vi "Autolab Complete Example (A).vi"() -> ()   [LabVIEW 2011]
uses:
  C:/Program Files/Metrohm Autolab/Autolab SDK 1.10/EcoChemie.Autolab.Sdk.dll
  EcoChemie.Autolab.Sdk.dll
panel:
  out "PotentialApplied":dbl
  in  "Abort":bool
  in  "fileName":string
  out "IsMeasuring":bool
  in  "Save":bool
  in  "start measure":bool
  in  "Stop":bool
  out "Value Y":dbl
  out "Value X":dbl
  out "XY Graph 2":cluster{"Y":dbl[], "Y":dbl[]}[](graph)
  in  "Signal X":string(combo)
  in  "Signal Y":string(combo)
  out "Setpoint":dbl
  out "Mode":i32(ring) items=["Potentiostatic", "Galvanostatic"]
  out "CurrentRange":i32(ring) items=["CR07_1A"=0, "CR06_10A"=1, "CR01_100A"=2, "CR00_1000A"=3, "CR05_20A"=20, "CR04_40A"=40, "CR03_50A"=60, "CR02_80A"=80, "CR19_1pA"=-12, "CR18_10pA"=-11, "CR17_100pA"=-10, "CR16_1nA"=-9, "CR15_10nA"=-8, "CR14_100nA"=-7, "CR13_1uA"=-6, "CR12_10uA"=-5, "CR11_100uA"=-4, "CR10_1mA"=-3, "CR09_10mA"=-2, "CR08_100mA"=-1]
  out "Bandwidth":i32(ring) items=["UltraHigh_Speed", "High_Speed", "High_Stability"]
  out "error out":errorcluster
  in  "Procedure":path=path "Standard Nova Procedures/Cyclic voltammetry.nox"
  in  "Load":bool
  in  "Hardware Setup File":path
  out "EI status supported for":string[](array[string])
  out "Oscillation":bool
  in  "Channel":i32(ring) items=["16"=15, "15"=14, "14"=13, "13"=12, "12"=11, "11"=10, "10"=9, "9"=8, "8"=7, "7"=6, "6"=5, "5"=4, "4"=3, "3"=2, "2"=1, "1"=0]
  out "IsConnected":bool
  out "Sample":dbl
  in  "usPerLoop 2":u16=20000
  in  "usPerLoop":u16=20000
  in  "Sampler Type":T1(ring)
  in  "Loops 2":i32=1 min=1
  in  "Loops":i32=1 min=1
  in  "Gain 2":i32(ring) items=["Gain_1"=0, "Gain_10"=64, "Gain_100"=128, "Gain_1000"=192]
  in  "Gain":i32(ring) items=["Gain_1"=0, "Gain_10"=64, "Gain_100"=128, "Gain_1000"=192]
  out "DIO Status P2 R":bool[](array[boolean])
  in  "DIO Status P2 W":bool[](array[boolean])
  in  "Port P2":i32(ring) items=["Port_A", "Port_B", "Port_C"]
  in  "P2 Direction":enum16{"Input(read)", "Output(write)"}(ring)
  out "DIO Status P1 R":bool[](array[boolean])
  in  "Port P1":i32(ring) items=["Port_A", "Port_B", "Port_C"]
  in  "P1 Direction":enum16{"Input(read)", "Output(write)"}(ring)
  in  "DIO Status P1 W":bool[](array[boolean])
  in  "voltage":dbl
  in  "channel":i32 min=0 max=16
  out "Value":dbl
  in  "Signal List":string(combo)
  out "Current":dbl
  out "Potential":dbl
  out "PotentialOverload":bool
  out "TemperatureOverload":bool
  out "CurrentOverload":bool
  out "ManualCellSwitch":bool
  out "Cell":bool
  in  "Setpoint":dbl
  in  "Current Range":i32(ring)=-3 items=["CR07_1A"=0, "CR06_10A"=1, "CR01_100A"=2, "CR00_1000A"=3, "CR05_20A"=20, "CR04_40A"=40, "CR03_50A"=60, "CR02_80A"=80, "CR19_1pA"=-12, "CR18_10pA"=-11, "CR17_100pA"=-10, "CR16_1nA"=-9, "CR15_10nA"=-8, "CR14_100nA"=-7, "CR13_1uA"=-6, "CR12_10uA"=-5, "CR11_100uA"=-4, "CR10_1mA"=-3, "CR09_10mA"=-2, "CR08_100mA"=-1]
  in  "Cell On/Off":i32(ring) items=["Off", "On"]
  in  "Bandwidth":i32(ring)=2 items=["UltraHigh_Speed", "High_Speed", "High_Stability"]
  in  "Mode":i32(ring) items=["Potentiostatic", "Galvanostatic"]
  in  "Embedded Exe File":path
  # "Create Autolab"
  # "Measuring"
  # "Electrochemical Interface"
  # "ADC"
  # "DIO"
  # "DAC"
  # "Sampler Signals"
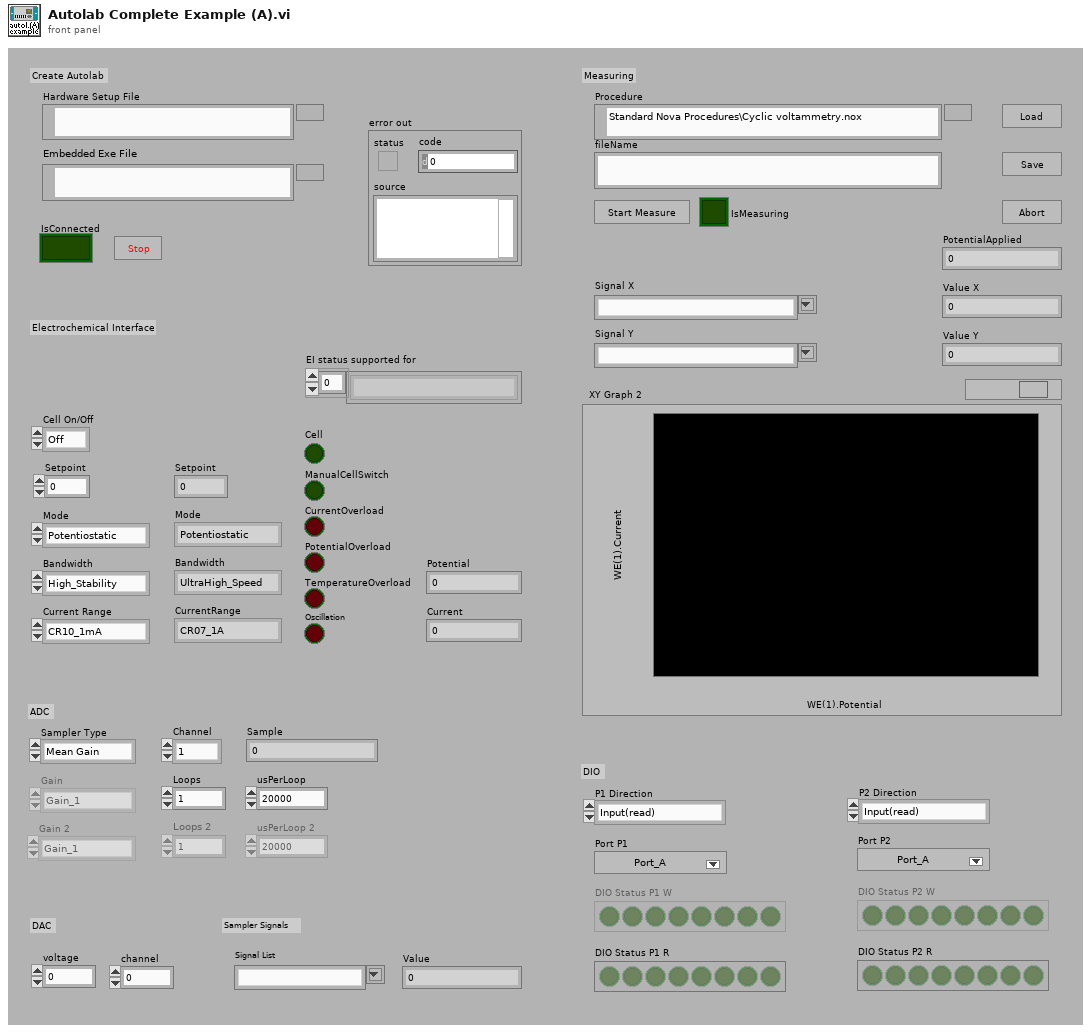
[diagram p1: front panel]
types:
  T1 = enum16{"Mean Gain", "Mean Fixed", "One Fixed", "One Gain"}
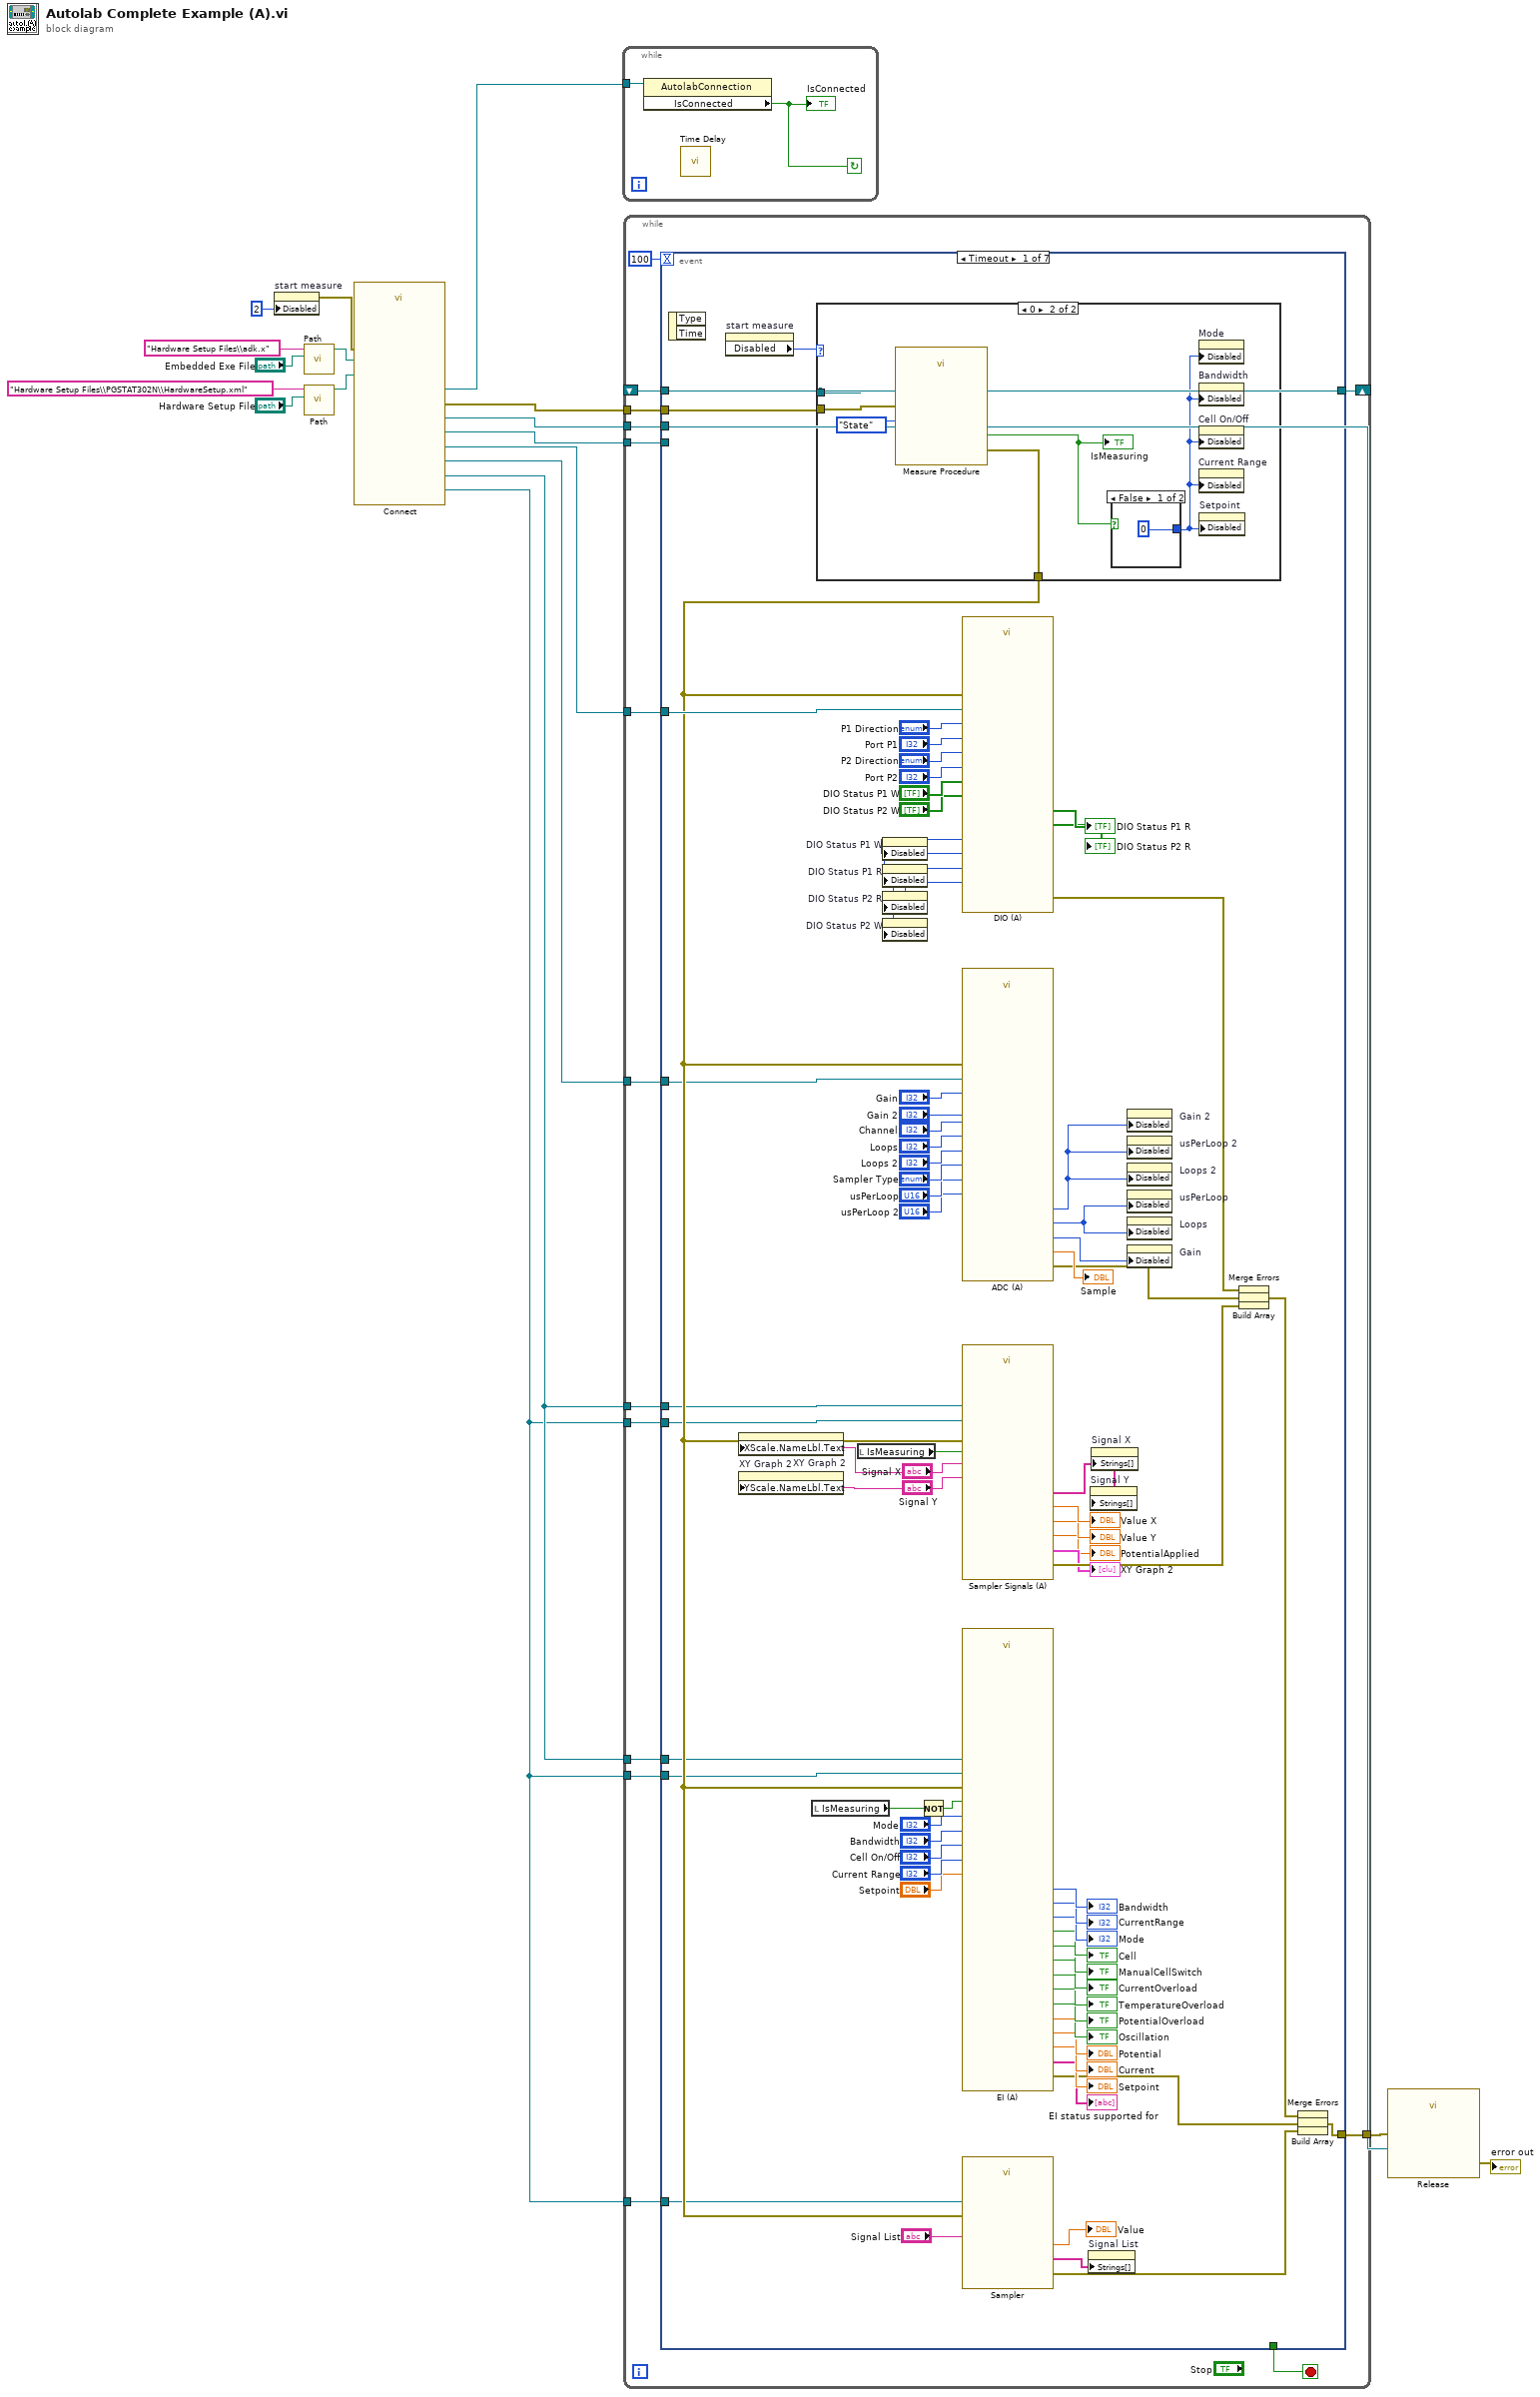
[diagram p0: block diagram]
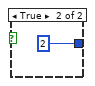
[diagram p3: hidden frame]
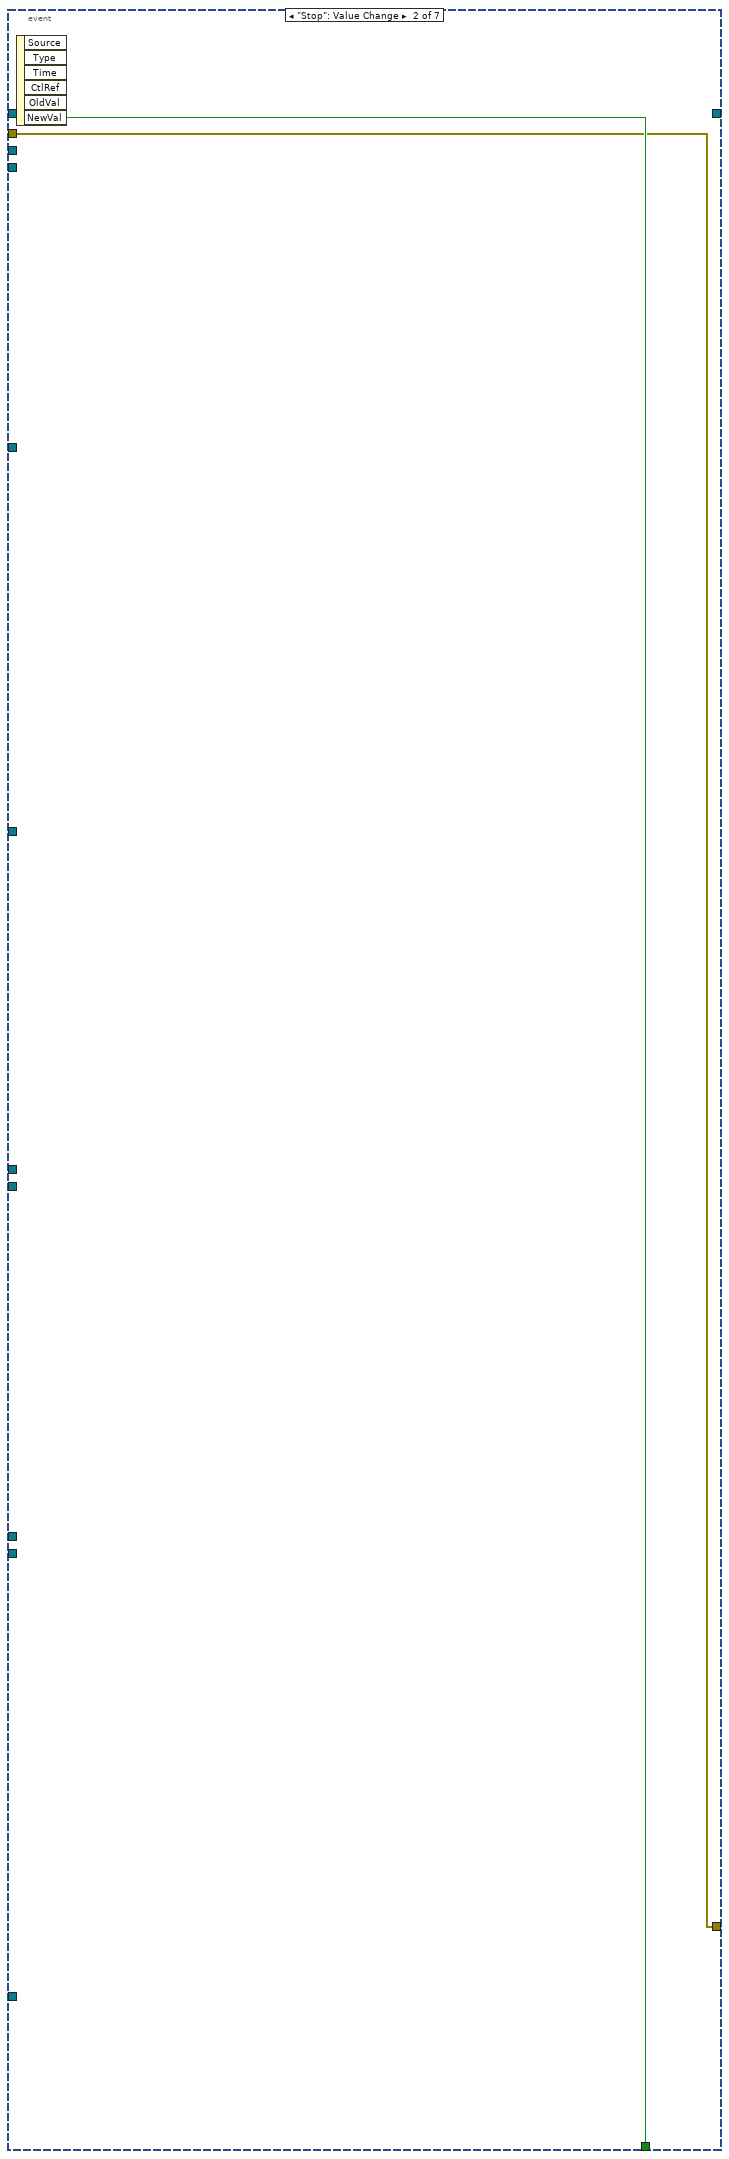
[diagram p4: hidden frame]
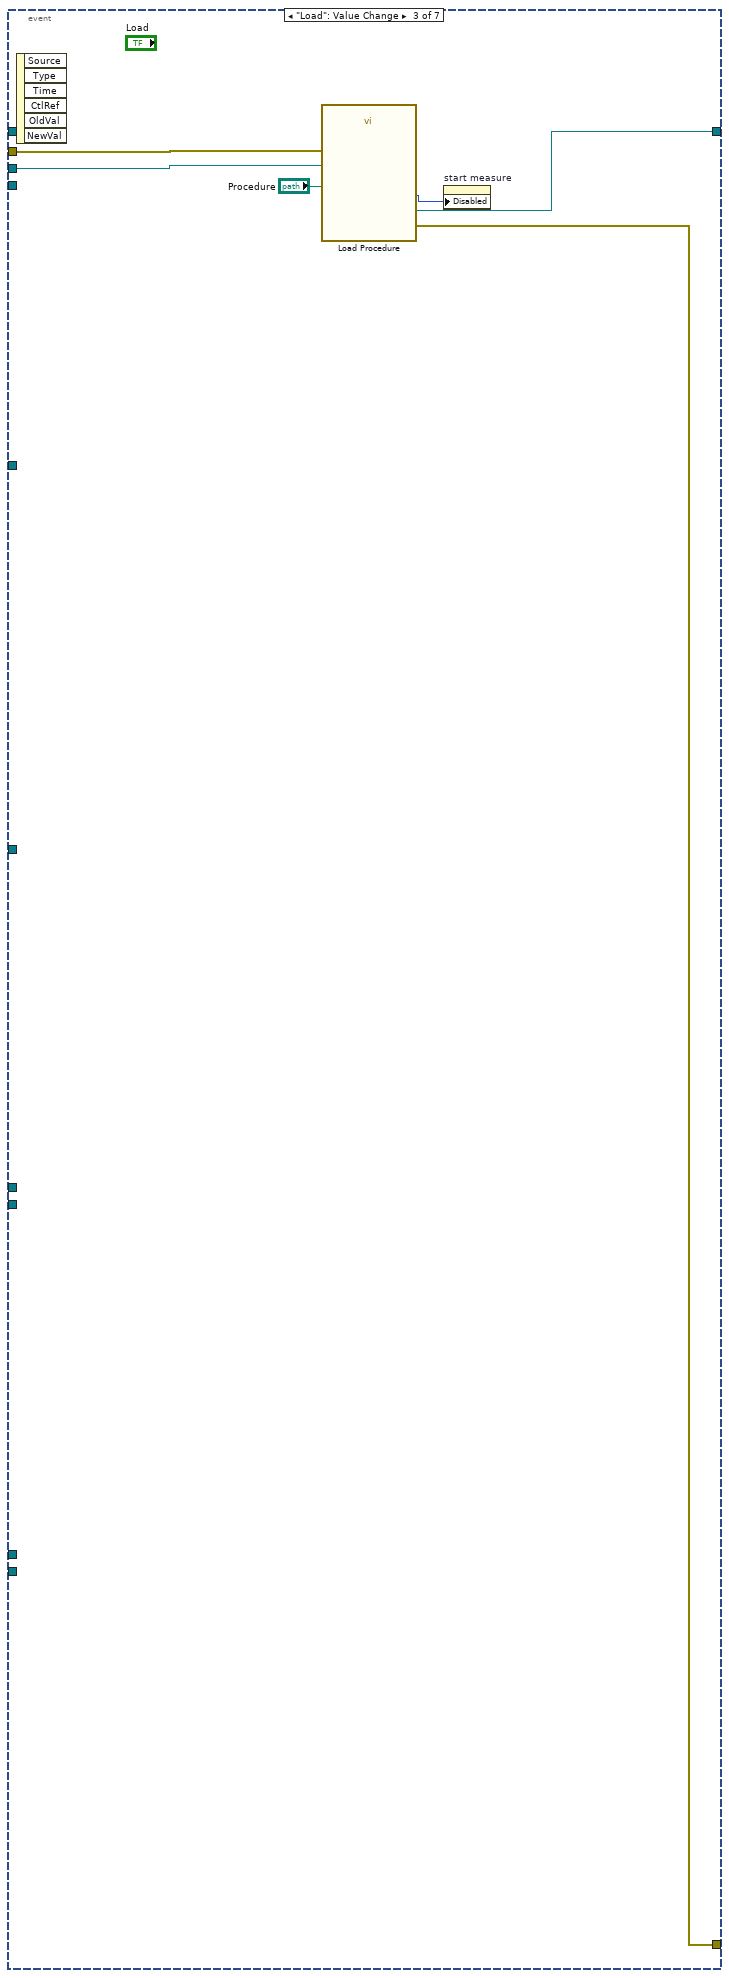
[diagram p5: hidden frame]
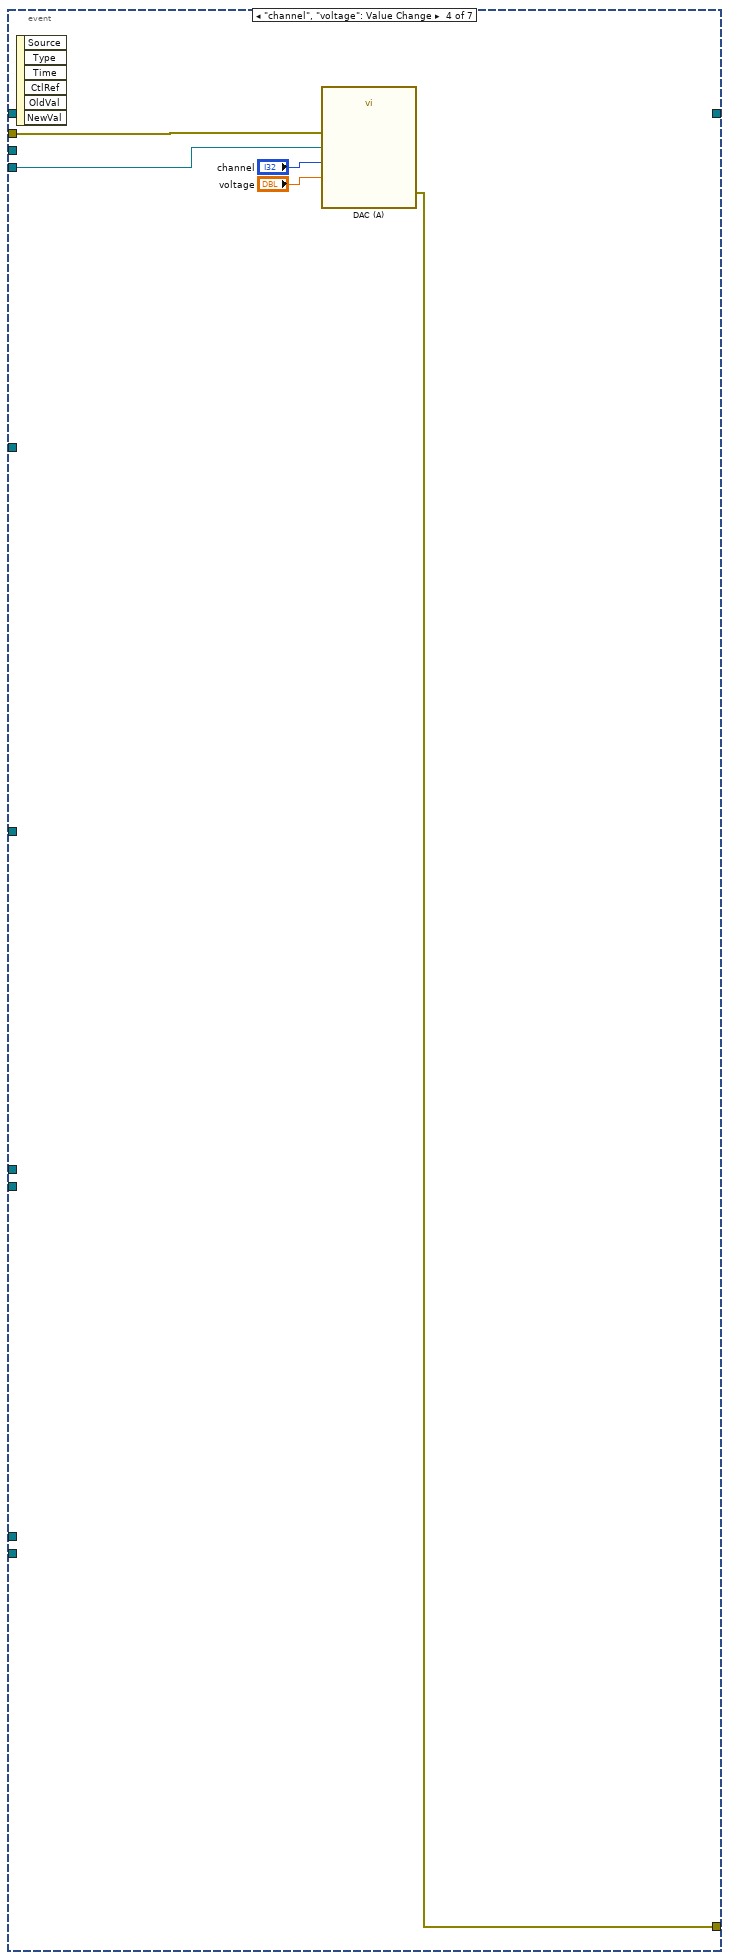
[diagram p6: hidden frame]
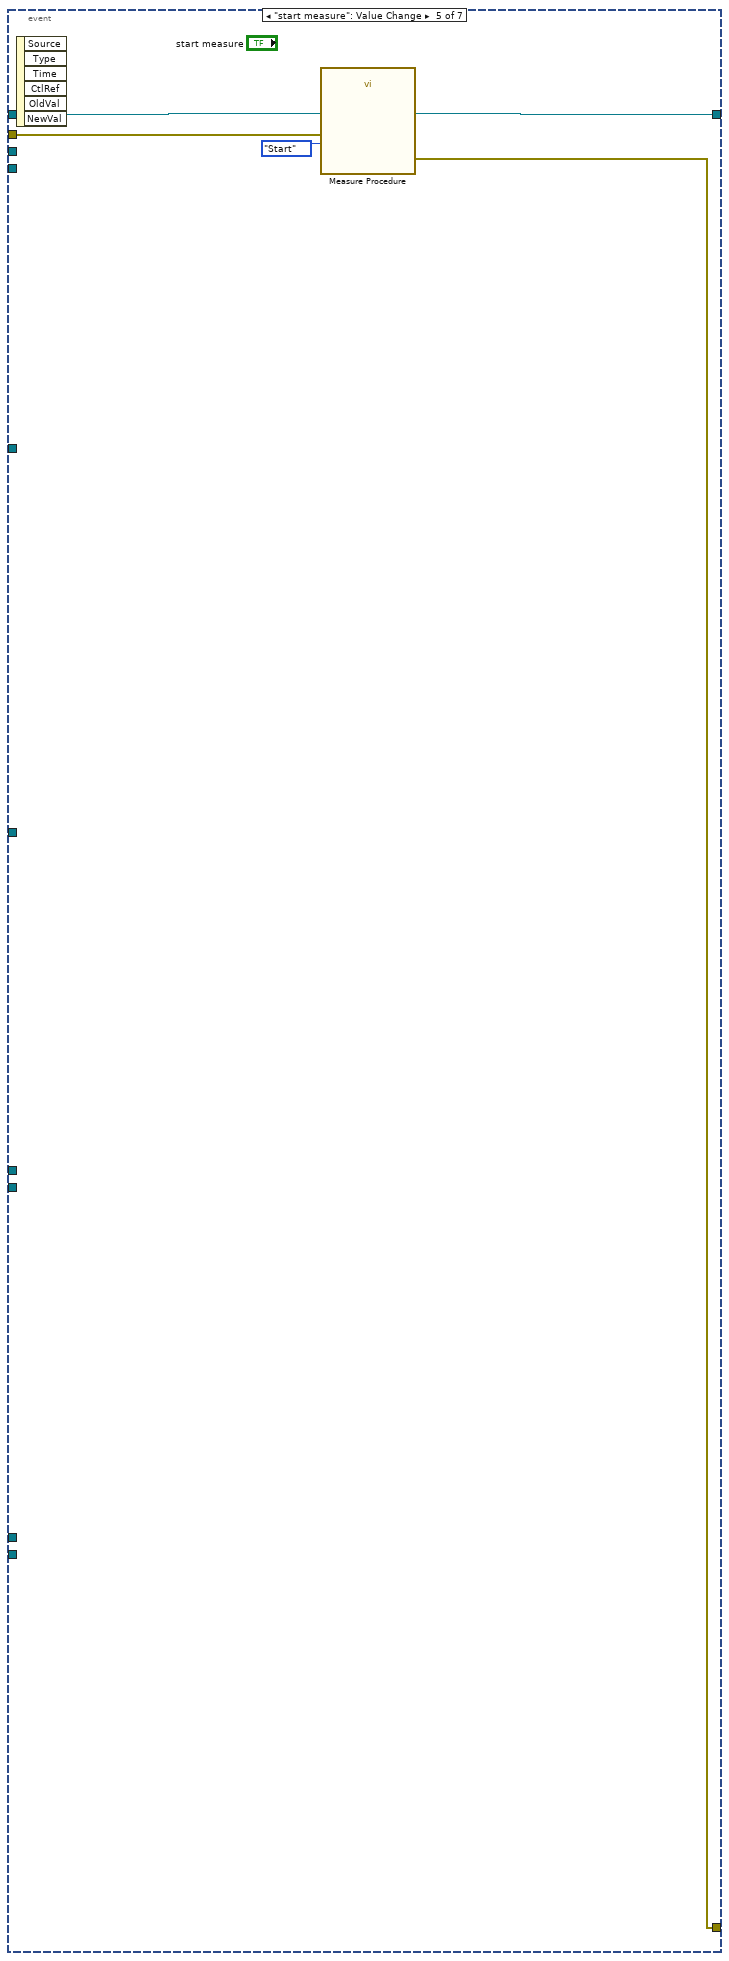
[diagram p7: hidden frame]
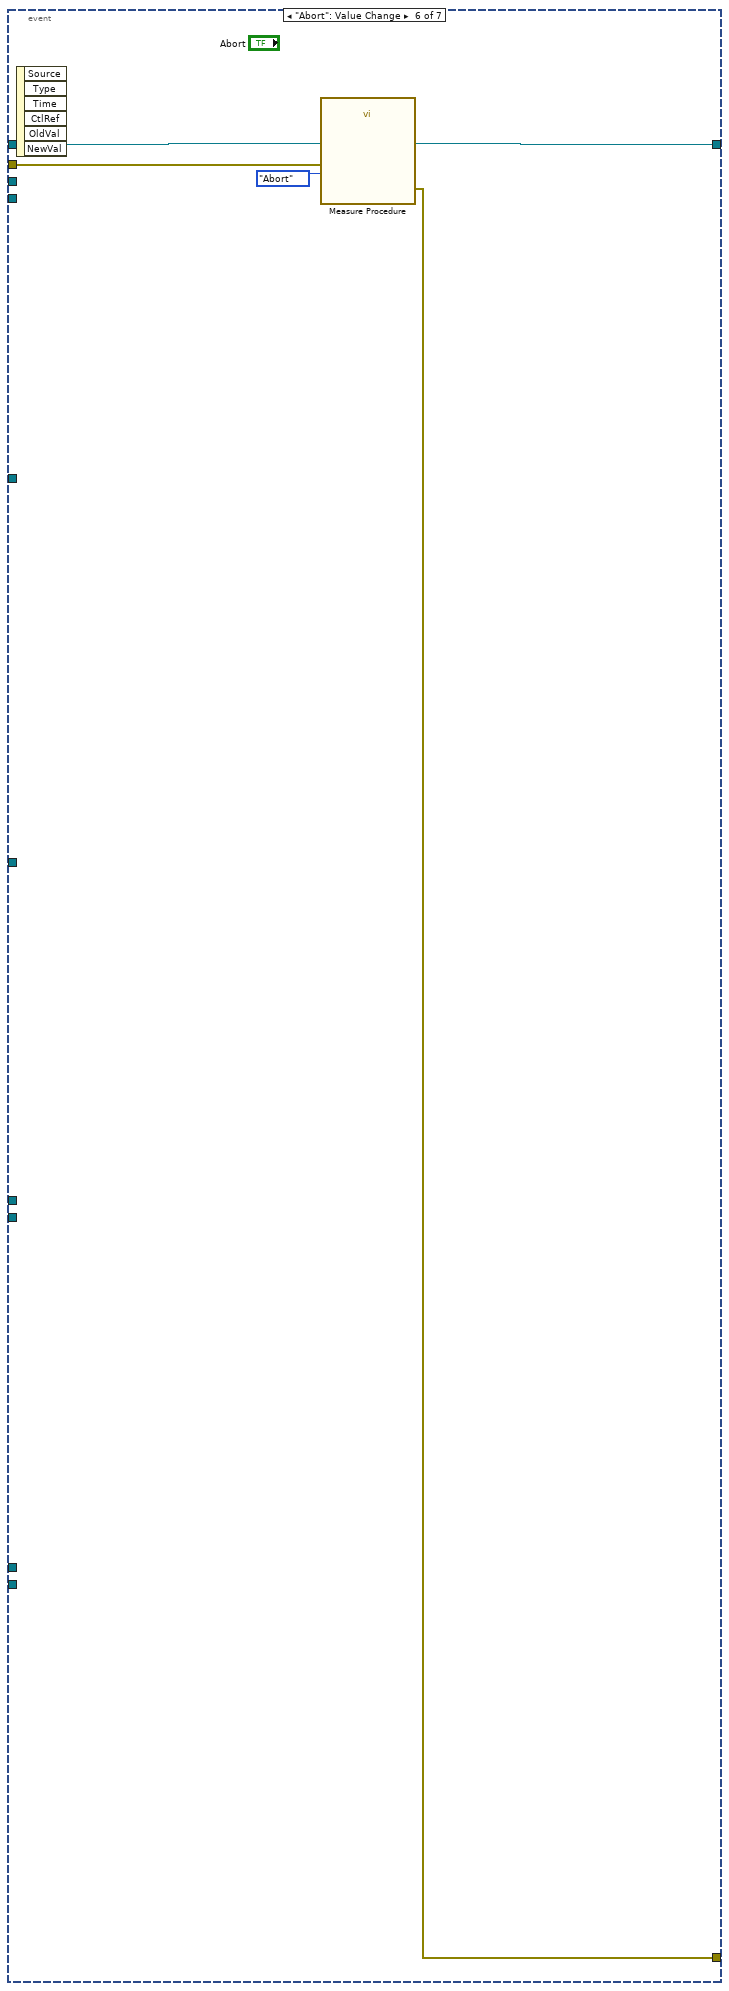
[diagram p8: hidden frame]
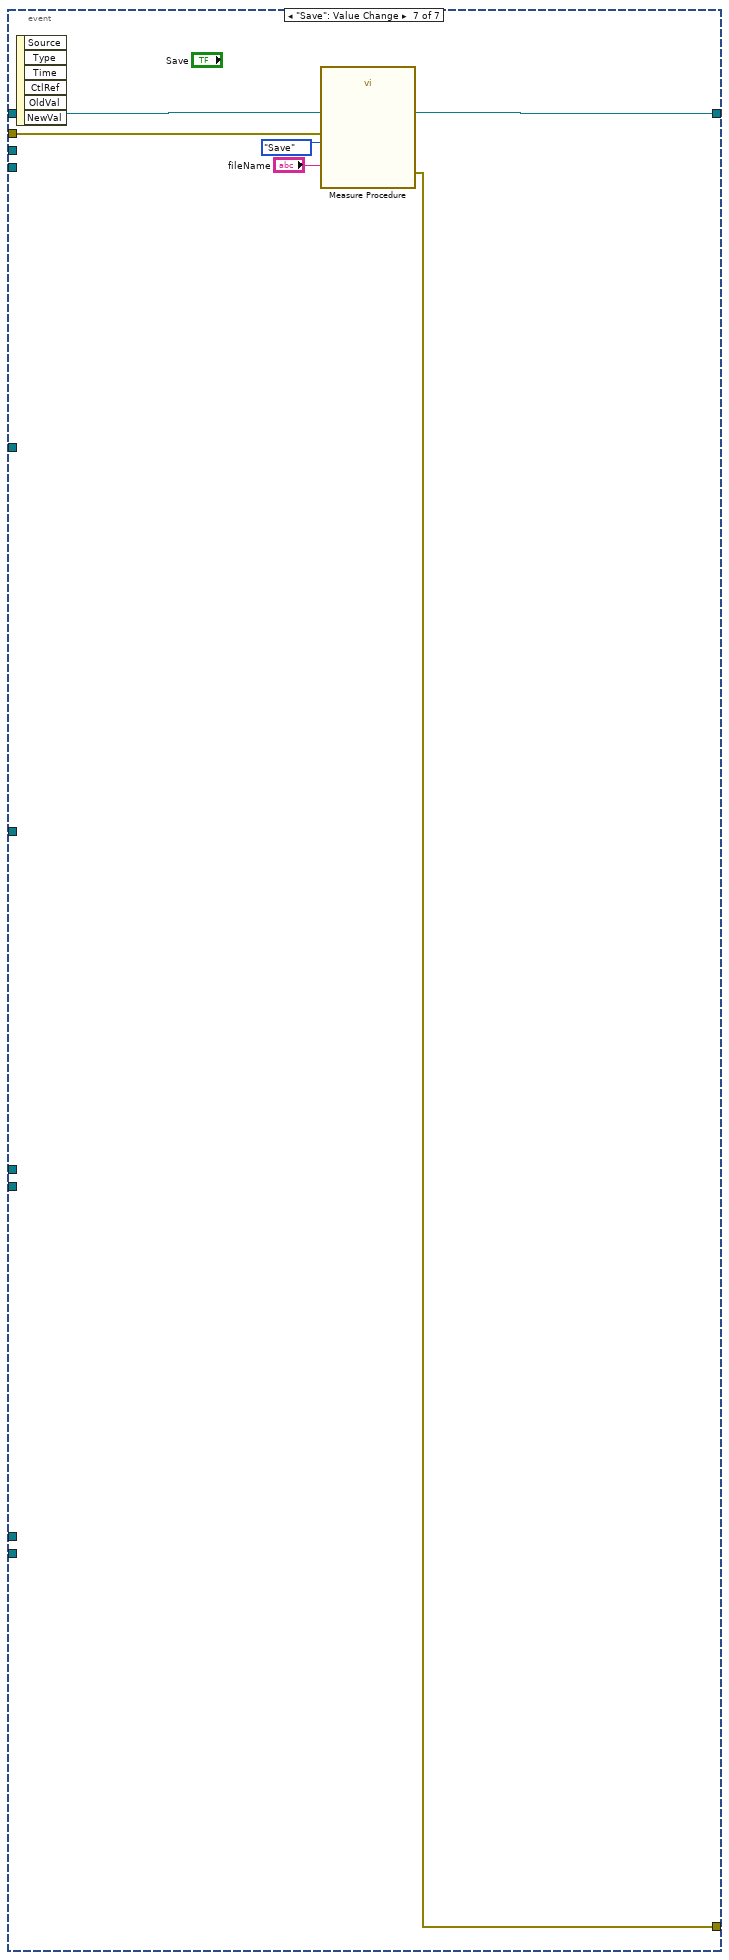
[diagram p9: hidden frame]
diagram:
  n1 = property on="start measure" class="Bool"("Disabled"=u8 2) -> (error out=w2:errorcluster)  [unwired: 2 in, 1 out]
  n2 = call "Path.vi"("File"="Embedded Exe File", "name or relative path"="Hardware Setup Files\\adk.x") -> ("appended path"=w5:path)  [unwired: 9 in]
  n3 = call "Path.vi"("File"="Hardware Setup File", "name or relative path"="Hardware Setup Files\\PGSTAT302N\\HardwareSetup.xml") -> ("appended path"=w6:path)  [unwired: 9 in]
  n4 = call "Connect.vi"("Embedded Exe File"=w5, "Hardware Setup File"=w6, "error in (no error)"=w2) -> ("Adc"=w13:refnum<k24>, "Dac"=w15:refnum<k24>, "Dio"=w14:refnum<k24>, "Sampler"=w11:refnum<k24>, "AutolabConnection"=w17:refnum<k24>, "instrument"=w9:refnum<k24>, "Ei"=w12:refnum<k24>, "error out"=w16:errorcluster)  [unwired: 5 in]
  n5 = while {
    tunnel: w17 -> [w20]
    stop <- w19 continue-if-true
    n6 = property class="AutolabConnection"(reference=w20) -> ("IsConnected"=w19:bool)  [unwired: 1 in, 2 out]
    "IsConnected" <- w19
    n7 = call "Time Delay"() -> ()  [unwired: 11 in, 1 out]
  }
  n8 = while {
    shift-right: [w32] -> _
    shift-left: _ -> [w33]
    tunnel: w16 -> [w31]
    tunnel: w9 -> [w30]
    tunnel: w15 -> [w29]
    tunnel: w14 -> [w28]
    tunnel: w13 -> [w27]
    tunnel: w11 -> [w26]
    tunnel: w12 -> [w25]
    tunnel: w11 -> [w24]
    tunnel: w11 -> [w23]
    tunnel: w12 -> [w22]
    tunnel: [w21] -> w10
    stop <- w35 stop-if-true
    n9 = event shown="[0] Timeout" {
      selector: _ -> [_ _ _ _ _ _ _]
      dyn-events: _ -> [_ _ _ _ _ _ _]
      timeout: 100 -> [_ _ _ _ _ _ _]
      tunnel: [_ w121 _ _ _ _ _] -> w35
      tunnel: w33 -> [w46 _ _ _ w135 w139 w143]
      tunnel: [w46 _ w125 _ w135 w139 w143] -> w32
      tunnel: w31 -> [w62 w120 w124 w129 w134 w138 w142]
      tunnel: w30 -> [_ _ w123 _ _ _ _]
      tunnel: w29 -> [_ _ _ w130 _ _ _]
      tunnel: w28 -> [w63 _ _ _ _ _ _]
      tunnel: w27 -> [w60 _ _ _ _ _ _]
      tunnel: w26 -> [w59 _ _ _ _ _ _]
      tunnel: w25 -> [w58 _ _ _ _ _ _]
      tunnel: w24 -> [w57 _ _ _ _ _ _]
      tunnel: w23 -> [w56 _ _ _ _ _ _]
      tunnel: w22 -> [w55 _ _ _ _ _ _]
      tunnel: [w48 w120 w122 w128 w133 w137 w141] -> w21
      event Timeout {
        n10 = event-data() -> ()  [unwired: 1 in, 2 out]
        n11 = property on="start measure" class="Bool"() -> ("Disabled"=w64:u8)  [unwired: 2 in, 2 out]
        n12 = property on="XY Graph 2" class="XYGraph (strict)"("XScale.NameLbl.Text"="Signal X") -> ()  [unwired: 2 in, 2 out]
        n13 = property on="XY Graph 2" class="XYGraph (strict)"("YScale.NameLbl.Text"="Signal Y") -> ()  [unwired: 2 in, 2 out]
        n14 = local read "IsMeasuring"() -> (w47:bool)
        n15 = case shown="0" w64 {
          tunnel: w46 -> [_ w114]
          tunnel: w62 -> [w111 w113]
          tunnel: [w111 w112] -> w61
          frame 2, Default {
          }
          frame 0 {
            n16 = call "Measure Procedure.vi"("error in"=w113, "Request for procedure"=enum16{"State", "Save", "Abort", "Start"}."State", "LoadProcedure"=w114) -> ("error out"=w112:errorcluster, "IsMeasuring"=w116:bool)  [unwired: 7 in]
            "IsMeasuring" <- w116
            n17 = case shown="False" w116 {
              tunnel: [u8 0 ("Disabled") u8 2 ("Disabled")] -> w117
              frame False {
              }
              frame True {
              }
            }
            n18 = property on="Mode" class="Ring (strict)"("Disabled"=w117) -> ()  [unwired: 2 in, 2 out]
            n19 = property on="Bandwidth" class="Ring (strict)"("Disabled"=w117) -> ()  [unwired: 2 in, 2 out]
            n20 = property on="Cell On/Off" class="Ring (strict)"("Disabled"=w117) -> ()  [unwired: 2 in, 2 out]
            n21 = property on="Current Range" class="Ring (strict)"("Disabled"=w117) -> ()  [unwired: 2 in, 2 out]
            n22 = property on="Setpoint" class="DigNum (strict)"("Disabled"=w117) -> ()  [unwired: 2 in, 2 out]
          }
        }
        n23 = local read "IsMeasuring"() -> (w43:bool)
        n24 = Not(x=w47) -> (.not. x?=w110:bool)
        n25 = call "DIO (A).vi"("Dio"=w63, "DIO Status P1 W"="DIO Status P1 W", "DIO Status P2 W"="DIO Status P2 W", "error in (no error)"=w61, "Port P1"="Port P1", "Port P2"="Port P2", "P1 Direction"="P1 Direction", "P2 Direction"="P2 Direction") -> ("Disable P1 W"=w80:u8, "Disable P2 W"=w77:u8, "DIO Status P1 R"=→"DIO Status P1 R":bool[], "Disable P1 R"=w79:u8, "DIO Status P2 R"=→"DIO Status P2 R":bool[], "Disable P2 R"=w78:u8, "error out"=w54:errorcluster)  [unwired: 5 in]
        n26 = property on="DIO Status P1 W" class="Arr (strict)"("Disabled"=w80) -> ()  [unwired: 2 in, 2 out]
        n27 = property on="DIO Status P1 R" class="Arr (strict)"("Disabled"=w79) -> ()  [unwired: 2 in, 2 out]
        n28 = property on="DIO Status P2 R" class="Arr (strict)"("Disabled"=w78) -> ()  [unwired: 2 in, 2 out]
        n29 = property on="DIO Status P2 W" class="Arr (strict)"("Disabled"=w77) -> ()  [unwired: 2 in, 2 out]
        n30 = call "ADC (A).vi"("Adc"=w60, "Loops 2"="Loops 2", "Gain"="Gain", "Loops"="Loops", "Sampler Type"="Sampler Type", "Gain 2"="Gain 2", "usPerLoop 2"="usPerLoop 2", "error in"=w61, "Channel"="Channel", "usPerLoop"="usPerLoop") -> ("Sample"=→"Sample":dbl, "Disable MeanGain"=w67:u8, "Disable MeanFixed"=w65:u8, "Disable OneFixed"=w66:u8, "error out"=w53:errorcluster)  [unwired: 1 in]
        n31 = call "Sampler Signals (A).vi"("IsMeasuring"=w43, "EI"=w55, "Sampler"=w59, "Signal X"="Signal X", "Signal Y"="Signal Y", "error in"=w61) -> ("PotentialApplied"=→"PotentialApplied":dbl, "X"=→"Value X":dbl, "Y"=→"Value Y":dbl, "XY Graph"=→"XY Graph 2":cluster{"Y":dbl[], "Y":dbl[]}[], "GetSignals"=w42:string[], "error out"=w52:errorcluster)  [unwired: 4 in]
        n32 = call "EI (A).vi"("Sampler"=w57, "Ei"=w58, "CellOnOff"="Cell On/Off", "Setpoint"="Setpoint", "Bandwidth"="Bandwidth", "CurrentRange"="Current Range", "Mode"="Mode", "error in (no error)"=w61, "Disable Sampler"=w110) -> ("Cell"=→"Cell":bool, "PotentialOverload"=→"PotentialOverload":bool, "ManualCellSwitch"=→"ManualCellSwitch":bool, "TemperatureOverload"=→"TemperatureOverload":bool, "CurrentOverload"=→"CurrentOverload":bool, "Oscillation"=→"Oscillation":bool, "Setpoint"=→"Setpoint":dbl, "Bandwidth"=→"Bandwidth":i32, "CurrentRange"=→"CurrentRange":i32, "Mode"=→"Mode":i32, "EI status supported for"=→"EI status supported for":string[], "Potential"=→"Potential":dbl, "Current"=→"Current":dbl, "error out"=w50:errorcluster)  [unwired: 5 in]
        n33 = call "Sampler.vi"("error in (no error)"=w61, "Signal List"="Signal List", "Sampler"=w56) -> ("error out"=w51:errorcluster, "Signal Value"=→"Value":dbl, "GetSignals"=w90:string[])  [unwired: 6 in]
        n34 = property on="Signal List" class="CmbBox"("Strings[]"=w90) -> ()  [unwired: 2 in, 2 out]
        n35 = property on="Signal Y" class="CmbBox"("Strings[]"=w42) -> ()  [unwired: 2 in, 2 out]
        n36 = property on="Signal X" class="CmbBox"("Strings[]"=w42) -> ()  [unwired: 2 in, 2 out]
        n37 = property on="Gain 2" class="Ring (strict)"("Disabled"=w65) -> ()  [unwired: 2 in, 2 out]
        n38 = property on="usPerLoop 2" class="DigNum (strict)"("Disabled"=w65) -> ()  [unwired: 2 in, 2 out]
        n39 = property on="Loops 2" class="DigNum (strict)"("Disabled"=w65) -> ()  [unwired: 2 in, 2 out]
        n40 = property on="usPerLoop" class="DigNum (strict)"("Disabled"=w67) -> ()  [unwired: 2 in, 2 out]
        n41 = property on="Loops" class="DigNum (strict)"("Disabled"=w67) -> ()  [unwired: 2 in, 2 out]
        n42 = property on="Gain" class="Ring (strict)"("Disabled"=w66) -> ()  [unwired: 2 in, 2 out]
        n43 = Build Array(w54, w53, w52) -> (w36:errorcluster[])
        n44 = Merge Errors(w36) -> (w49:errorcluster)
        n45 = Build Array(w49, w50, w51) -> (w37:errorcluster[])
        n46 = Merge Errors(w37) -> (w48:errorcluster)
      }
      event "Stop": Value Change {
        n47 = event-data() -> ("NewVal"=w121:bool)  [unwired: 1 in, 5 out]
      }
      event "Load": Value Change {
        n48 = event-data() -> ()  [unwired: 1 in, 6 out]
        n49 = call "Load Procedure.vi"("error in (no error)"=w124, "Procedure"="Procedure", "Instrument"=w123) -> ("error out"=w122:errorcluster, "Numeric"=w127:i32, "LoadProcedure"=w125:refnum<k24>)  [unwired: 5 in, 1 out]
        n50 = property on="start measure" class="Bool"("Disabled"=w127) -> ()  [unwired: 2 in, 2 out]
      }
      event "channel", "voltage": Value Change {
        n51 = event-data() -> ()  [unwired: 1 in, 6 out]
        n52 = call "DAC (A).vi"("error in (no error)"=w129, "voltage"="voltage", "channel"="channel", "Dac"=w130) -> ("error out"=w128:errorcluster)  [unwired: 7 in]
      }
      event "start measure": Value Change {
        n53 = event-data() -> ()  [unwired: 1 in, 6 out]
        n54 = call "Measure Procedure.vi"("error in"=w134, "Request for procedure"=enum16{"State", "Save", "Abort", "Start"}."Start", "LoadProcedure"=w135) -> ("error out"=w133:errorcluster)  [unwired: 7 in, 1 out]
      }
      event "Abort": Value Change {
        n55 = event-data() -> ()  [unwired: 1 in, 6 out]
        n56 = call "Measure Procedure.vi"("error in"=w138, "Request for procedure"=enum16{"State", "Save", "Abort", "Start"}."Abort", "LoadProcedure"=w139) -> ("error out"=w137:errorcluster)  [unwired: 7 in, 1 out]
      }
      event "Save": Value Change {
        n57 = event-data() -> ()  [unwired: 1 in, 6 out]
        n58 = call "Measure Procedure.vi"("error in"=w142, "fileName"="fileName", "Request for procedure"=enum16{"State", "Save", "Abort", "Start"}."Save", "LoadProcedure"=w143) -> ("error out"=w141:errorcluster)  [unwired: 6 in, 1 out]
      }
    }
  }
  n59 = call "Release.vi"("error in (no error)"=w10, "Instrument"=w9) -> ("error out"=→"error out":errorcluster)  [unwired: 9 in]
